vi "ReportPart_A131258.vi"(6 "试验项目":enum32{"左工位", "右工位"}(ring), 8 "error in":errorcluster, 9 "索引":i32, 10 "合格":T1, 11 "report in":refnum<class "NI_report.lvclass">) -> (0 "error out 2":errorcluster caption="error out", 2 "索引OUT":i32, 3 "report out":refnum<class "NI_report.lvclass">)   [LabVIEW 2020]
uses:
  <vilib>/Utility/NIReport.llb/NI_report.lvclass
  OK.ctl
  <vilib>/Utility/NIReport.llb/image depth.ctl
  <vilib>/addons/_office/_exclsub.llb/font.ctl
  Global_Variable/A131258.vi
  Global_Variable/Global.vi
  <vilib>/Utility/NIReport.llb/Append Report Text (str wrap).vi
  <vilib>/addons/_office/word.llb/Word Easy Table (str).vi
  <vilib>/Utility/NIReport.llb/NI_ReportGenerationCore.lvlib
  <vilib>/Utility/NIReport.llb/Word/NI_Word.lvclass
  <vilib>/addons/_office/NI_ReportGenerationToolkit.lvlib
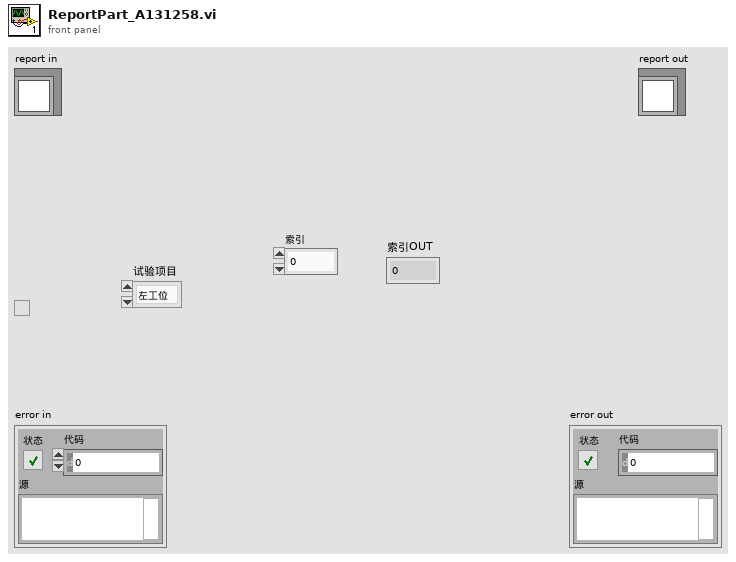
[diagram p1: front panel]
types:
  T1 = typedef "OK.ctl" = bool
  T2 = cluster{"Charset (-1)":i16, "Weight (-1)":i16, "Name":string, "Size":string}
  T3 = cluster{"Italic":enum16{"Italic Unchanged", "Italic On", "Italic Off"}, "Strike Through":enum16{"Strike Through Unchanged", "Strike Through On", "Strike Through Off"}, "Underline":enum16{"Underline Unchanged", "Underline On", "Underline Off"}, "Bold":enum16{"Bold Unchanged", "Bold On", "Bold Off"}}
  T4 = typedef "NI_ReportGenerationToolkit.lvlib/font.ctl" = cluster{"font name":string, "font size":dbl, "bold":u16, "italic":u16, "underline":u16, "strike through":u16, "font color":u32}
  T5 = typedef "NI_ReportGenerationCore.lvlib/image depth.ctl" = u16
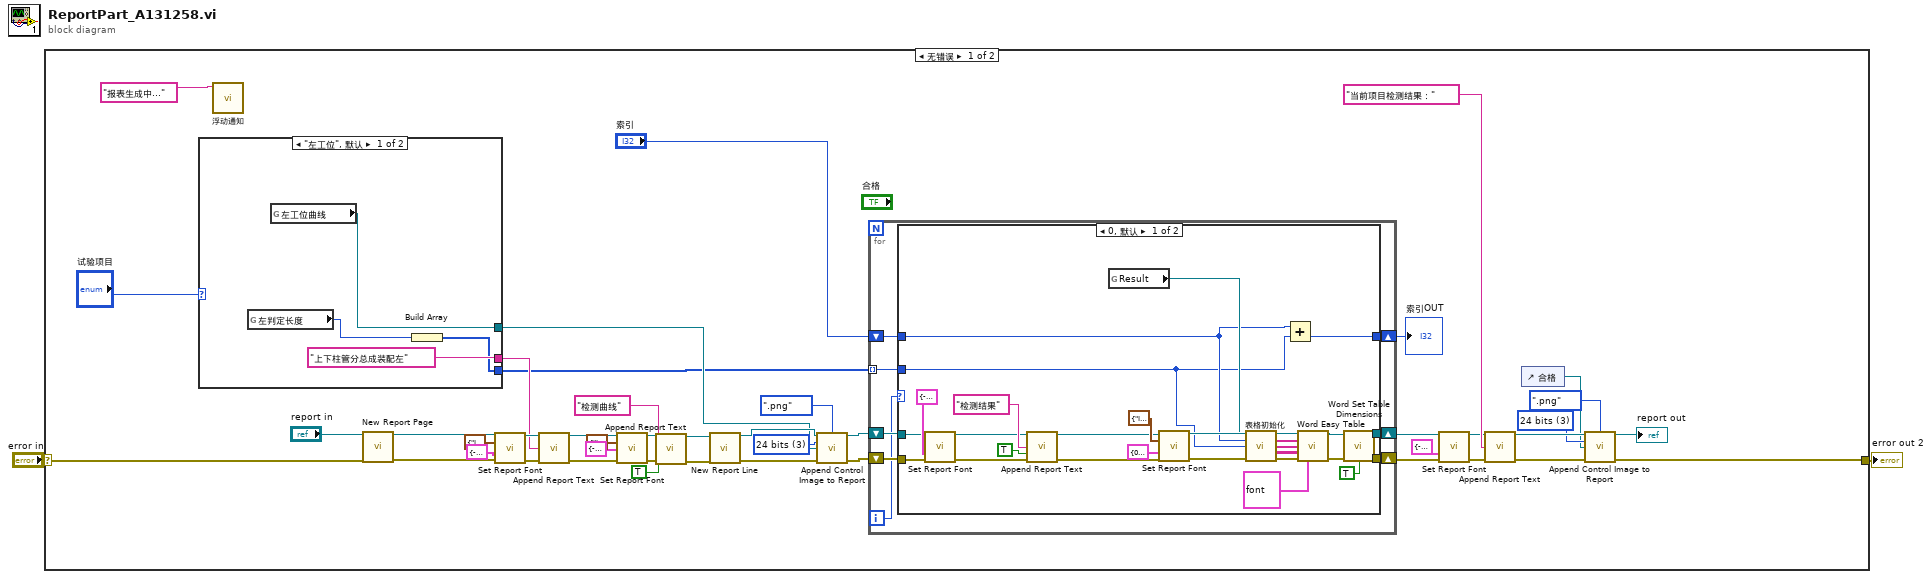
[diagram p0: block diagram]
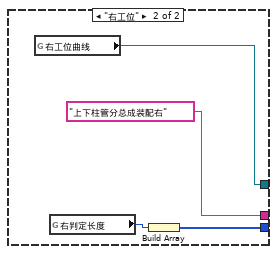
[diagram p3: hidden frame]
diagram:
  n1 = case shown="无错误" "error in" {
    selector: "error in" -> [w25 w93]
    tunnel: [w19 w93] -> w1
    frame No Error {
      w17 = T5 3 items=["B&W", "4 bits", "8 bits", "24 bits"] ("image depth")
      w44 = T5 3 items=["B&W", "4 bits", "8 bits", "24 bits"] ("image depth")
      n2 = case shown="\"左工位\", 默认" "试验项目" {
        tunnel: [w87 w90] -> w8
        tunnel: ["上下柱管分总成装配左" ("text") "上下柱管分总成装配右" ("text")] -> w38
        tunnel: [w85 w89] -> w7
        frame "左工位", Default {
          n3 = global read "Global.vi" "左判定长度"() -> (w86:i32)
          n4 = global read "A131258.vi" "左工位曲线"() -> (w87:refnum<vi>)
          n5 = Build Array(w86) -> (w85:i32[])
        }
        frame "右工位" {
          n6 = global read "A131258.vi" "右工位曲线"() -> (w90:refnum<vi>)
          n7 = global read "Global.vi" "右判定长度"() -> (w91:i32)
          n8 = Build Array(w91) -> (w89:i32[])
        }
      }
      n9 = call "浮动通知.vi"("通知内容"="报表生成中...") -> ()  [unwired: 11 in]
      n10 = call-dynamic "New Report Page.vi"("report in"="report in", "error in (no error)"=w25) -> ("report out"=w23:refnum<class "NI_report.lvclass">, "error out"=w24:errorcluster)  [unwired: 12 in]
      n11 = call-dynamic "Set Report Font.vi"("report in"=w23, "text options"=T3 {"Italic"=enum."Italic Unchanged", "Strike Through"=enum."Strike Through Unchanged", "Underline"=enum."Underline Unchanged", "Bold"=enum."Bold On"}, "font settings"=T2 {"Charset (-1)"=-1, "Weight (-1)"=-1, "Name"="楷体", "Size"="16 "}, "error in (no error)"=w24) -> ("report out"=w43:refnum<class "NI_report.lvclass">, "error out"=w42:errorcluster)  [unwired: 9 in, 1 out]
      n12 = call-poly <vilib>:"Append Report Text.vi"("report in"=w43, "text"=w38, "error in (no error)"=w42) -> ("report out"=w36:refnum<class "NI_report.lvclass">, "error out"=w35:errorcluster)  [unwired: 9 in, 2 out]
      n13 = call-dynamic "Set Report Font.vi"("report in"=w36, "text options"=T3 {"Italic"=enum."Italic Unchanged", "Strike Through"=enum."Strike Through Unchanged", "Underline"=enum."Underline Unchanged", "Bold"=enum."Bold Off"}, "font settings"=T2 {"Charset (-1)"=-1, "Weight (-1)"=-1, "Name"="宋体", "Size"="12 "}, "error in (no error)"=w35) -> ("report out"=w32:refnum<class "NI_report.lvclass">, "error out"=w29:errorcluster)  [unwired: 9 in, 1 out]
      n14 = call-poly <vilib>:"Append Report Text.vi"("report in"=w32, "text"="检测曲线", "append on new line? (F)"=TRUE, "error in (no error)"=w29) -> ("report out"=w31:refnum<class "NI_report.lvclass">, "error out"=w30:errorcluster)  [unwired: 8 in, 2 out]
      n15 = call-dynamic "New Report Line.vi"("report in"=w31, "error in (no error)"=w30) -> ("report out"=w45:refnum<class "NI_report.lvclass">, "error out"=w46:errorcluster)  [unwired: 12 in]
      n16 = call-dynamic "Append Control Image to Report.vi"("report in"=w45, "image file type (.jpg)"=enum16{".jpg", ".png"}.".png", "image depth"=w44, "ctrl reference"=w8, "error in (no error)"=w46) -> ("report out"=w40:refnum<class "NI_report.lvclass">, "error out"=w39:errorcluster)  [unwired: 7 in, 2 out]
      n17 = for {
        tunnel: w7 -> [w50] mode=indexing
        shift-right: [w52] -> w10
        shift-left: w40 -> [w54]
        shift-right: [w51] -> w9
        shift-left: w39 -> [w53]
        shift-right: [w47] -> w4
        shift-left: "索引" -> [w48]
        i -> [w49]
        n18 = case shown="0, 默认" w49 {
          tunnel: w54 -> [w77 w84]
          tunnel: w53 -> [w75 w83]
          tunnel: [w62 w84] -> w52
          tunnel: [w61 w83] -> w51
          tunnel: w50 -> [w55 _]
          tunnel: w48 -> [w56 w82]
          tunnel: [w57 w82] -> w47
          frame 0, Default {
            n19 = call-dynamic "Set Report Font.vi"("report in"=w77, "font settings"=T2 {"Charset (-1)"=-1, "Weight (-1)"=-1, "Name"="宋体", "Size"="12 "}, "error in (no error)"=w75) -> ("report out"=w78:refnum<class "NI_report.lvclass">, "error out"=w76:errorcluster)  [unwired: 10 in, 1 out]
            n20 = call-poly <vilib>:"Append Report Text.vi"("report in"=w78, "text"="检测结果", "append on new line? (F)"=TRUE, "error in (no error)"=w76) -> ("report out"=w60:refnum<class "NI_report.lvclass">, "error out"=w59:errorcluster)  [unwired: 8 in, 2 out]
            n21 = global read "Global.vi" "Result"() -> (w58:refnum<vi>)
            n22 = call-dynamic "Set Report Font.vi"("report in"=w60, "text options"=T3 {"Italic"=enum."Italic Unchanged", "Strike Through"=enum."Strike Through Unchanged", "Underline"=enum."Underline Unchanged", "Bold"=enum."Bold Unchanged"}, "font settings"=T2 {"Charset (-1)"=0, "Weight (-1)"=-1, "Name"="微软雅黑", "Size"="12 "}, "error in (no error)"=w59) -> ("report out"=w64:refnum<class "NI_report.lvclass">, "error out"=w63:errorcluster)  [unwired: 9 in, 1 out]
            n23 = call "表格初始化.vi"("表格引用"=w58, "索引"=w56, "长度"=w55, "错误输入（无错误）"=w63) -> ("行首字符串[]"=w66:string[], "列首字符串[]"=w65:string[], "文本数据"=w68:string[][], "错误输出"=w71:errorcluster)  [unwired: 7 in, 1 out]
            n24 = Add(x=w56, y=w55) -> (x+y=w57:i32)
            n25 = call-poly <vilib>:"Word Easy Table.vi"("report in"=w64, "row headers"=w66, "column headers"=w65, "data"=w68, "error in (no error)"=w71, "font"=T4 {"font name"="宋体", "font size"=12.0, "bold"=2, "italic"=2, "underline"=2, "strike through"=2, "font color"=16777216}) -> ("report out"=w69:refnum<class "NI_report.lvclass">, "error out"=w70:errorcluster)  [unwired: 7 in, 1 out]
            n26 = call <vilib>:"Word Set Table Dimensions.vi"("report in"=w69, "error in (no error)"=w70, "fit to page width? (F)"=TRUE) -> ("report out"=w62:refnum<class "NI_report.lvclass">, "error out"=w61:errorcluster)  [unwired: 11 in]
          }
          frame -1 {
          }
        }
      }
      "索引OUT" <- w4
      n27 = call-dynamic "Set Report Font.vi"("report in"=w10, "font settings"=T2 {"Charset (-1)"=-1, "Weight (-1)"=-1, "Name"="宋体", "Size"="16 "}, "error in (no error)"=w9) -> ("report out"=w14:refnum<class "NI_report.lvclass">, "error out"=w15:errorcluster)  [unwired: 10 in, 1 out]
      n28 = call-poly <vilib>:"Append Report Text.vi"("report in"=w14, "text"="当前项目检测结果：", "error in (no error)"=w15) -> ("report out"=w22:refnum<class "NI_report.lvclass">, "error out"=w20:errorcluster)  [unwired: 9 in, 2 out]
      n29 = control-ref of="合格"() -> (w16:refnum<vi>)
      n30 = call-dynamic "Append Control Image to Report.vi"("report in"=w22, "image file type (.jpg)"=enum16{".jpg", ".png"}.".png", "image depth"=w17, "ctrl reference"=w16, "error in (no error)"=w20) -> ("report out"=→"report out":refnum<class "NI_report.lvclass">, "error out"=w19:errorcluster)  [unwired: 7 in, 2 out]
    }
    frame Error {
    }
  }
  "error out 2" <- w1
